vi "RunEXE.vi"(0 "EXE Path":path, 11 "error in (no error)":errorcluster) -> (4 "Application Ref":refnum<vi>, 15 "error out":errorcluster)   [LabVIEW 2016, in "Drona.lvlib"]
doc: "Launches EXE and returns an application reference for the given EXE path"
uses:
  Drona.lvlib
  <vilib>/Utility/config.llb/Read Key (I32).vi
  <vilib>/SLL Toolkit/SLL File IO/SLL File IO.lvlib
  <vilib>/Utility/config.llb/NI_LVConfig.lvlib
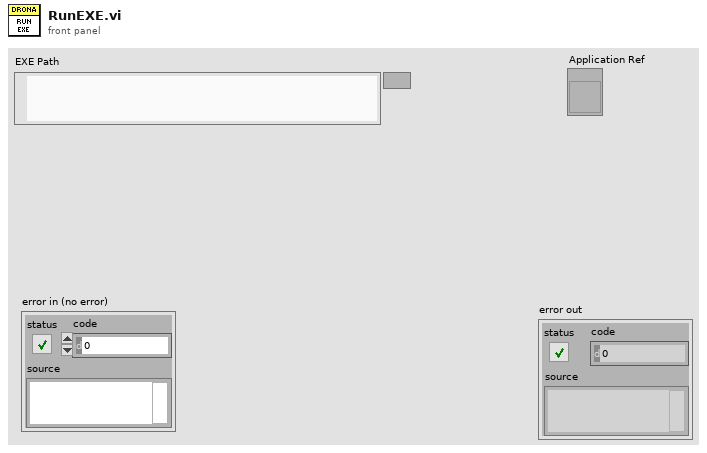
[diagram p1: front panel]
types:
  T1 = typedef "NI_LVConfig.lvlib/Config Data RefNum.ctl" = refnum<k1>
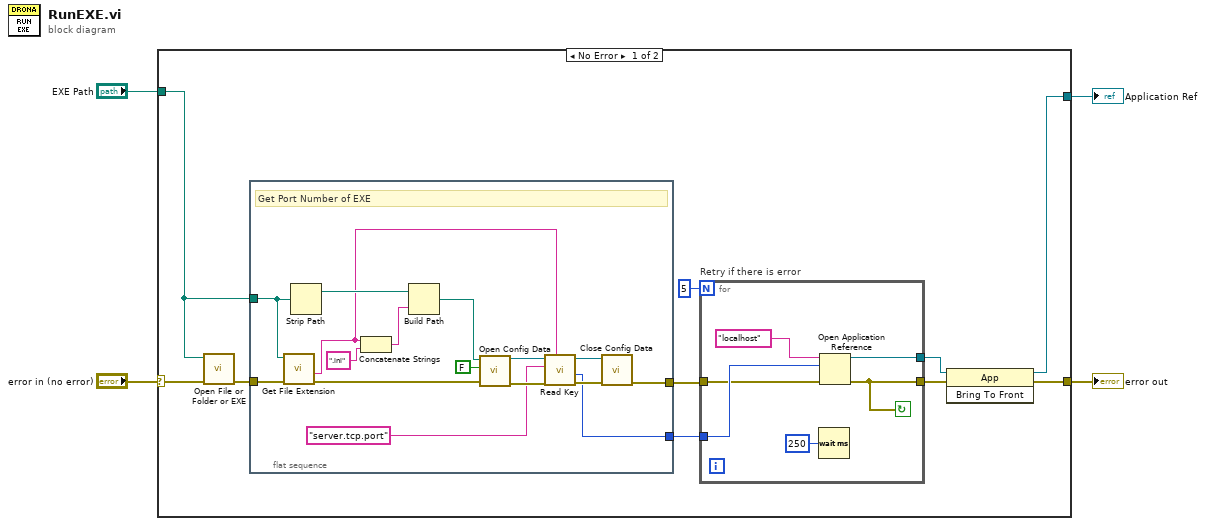
[diagram p0: block diagram]
diagram:
  n1 = case shown="No Error" "error in (no error)" {
    selector: "error in (no error)" -> [w14 w37]
    tunnel: [w9 w37] -> w3
    tunnel: [w6 _] -> w2
    tunnel: "EXE Path" -> [w12 _]
    frame No Error {
      n2 = call <vilib>:"Open File or Folder or EXE.vi"("error in (no error)"=w14, "Path"=w12) -> ("error out"=w13:errorcluster)  [unwired: 9 in]
      n3 = flat-sequence {
        tunnel: w13 -> [w30]
        tunnel: w12 -> [w29]
        tunnel: [w17] -> w11
        tunnel: [w16] -> w10
        frame #0 {
          # "Get Port Number of EXE"
          n4 = call <vilib>:"Get File Extension.vi"("error in (no error)"=w30, "file"=w29) -> ("error out"=w15:errorcluster, "filename without extension"=w21:string)  [unwired: 5 in, 3 out]
          n5 = Strip Path(path=w29) -> (stripped path=w27:path)  [unwired: 1 out]
          n6 = Concatenate Strings(w21, ".ini" ("string")) -> (w26:string)
          n7 = Build Path(base path=w27, name or relative path=w26) -> (appended path=w25:path)
          n8 = call <vilib>:"Open Config Data.vi"("error in (no error)"=w15, "create file if necessary (T)"=FALSE, "configuration file path"=w25) -> ("error out"=w22:errorcluster, "refnum"=w23:T1)  [unwired: 6 in, 1 out]
          n9 = call-poly <vilib>:"Read Key.vi"("section"=w21, "error in (no error)"=w22, "key"="server.tcp.port", "refnum"=w23) -> ("error out"=w19:errorcluster, "value"=w17:i32, "refnum out"=w18:T1)  [unwired: 4 in, 1 out]
          n10 = call <vilib>:"Close Config Data.vi"("error in (no error)"=w19, "refnum"=w18) -> ("error out"=w16:errorcluster)  [unwired: 8 in, 1 out]
        }
      }
      n11 = for "Retry if there is error" {
        N: 5 -> [_]
        tunnel: w11 -> [w36]
        tunnel: [w33] -> w7
        tunnel: w10 -> [w35]
        tunnel: [w31] -> w8
        stop <- w31 continue-if-true
        n12 = Wait (ms)(milliseconds to wait=u32 250) -> ()  [unwired: 1 out]
        n13 = Open Application Reference(8:w35, 10:w36, 11:"localhost" ("machine name (\"\":  open local reference)")) -> (0:w31:errorcluster, 3:w33:refnum<vi>)  [unwired: 1 in]
      }
      n14 = invoke class="App" method="Bring To Front"(reference=w7, error in=w8) -> (reference out=w6:refnum<vi>, error out=w9:errorcluster)  [unwired: 1 in, 1 out]
    }
    frame Error {
    }
  }
  "error out" <- w3
  "Application Ref" <- w2
